vi "verify unique value in a list.vi"(7 "parameter name":string, 8 "error in (no error)":errorcluster, 9 "value":u16, 10 "list of values":u16[](array[numeric]), 11 "Simulated_CCD_Camera in":refnum<class "Simulated_CCD_Camera.lvclass">) -> (0 "error out":errorcluster, 3 "Simulated_CCD_Camera out":refnum<class "Simulated_CCD_Camera.lvclass">)   [LabVIEW 2018, in "Simulated_CCD_Camera.lvclass"]
uses:
  Simulated_CCD_Camera.lvclass
  Simulated_CCD_Camera.lvclass/Simulated_CCD_Camera.ctl
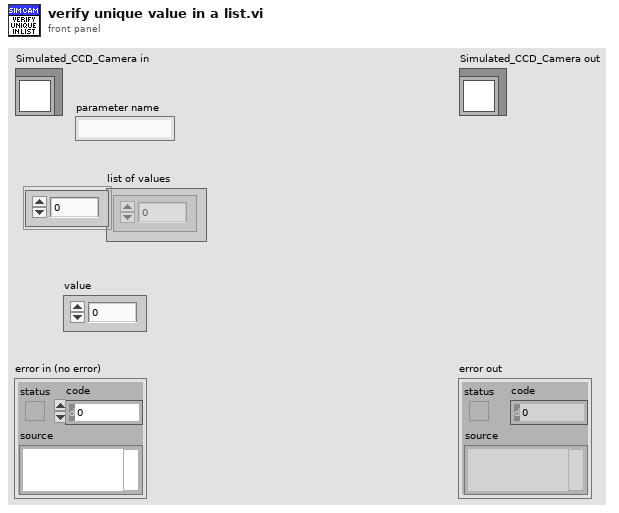
[diagram p1: front panel]
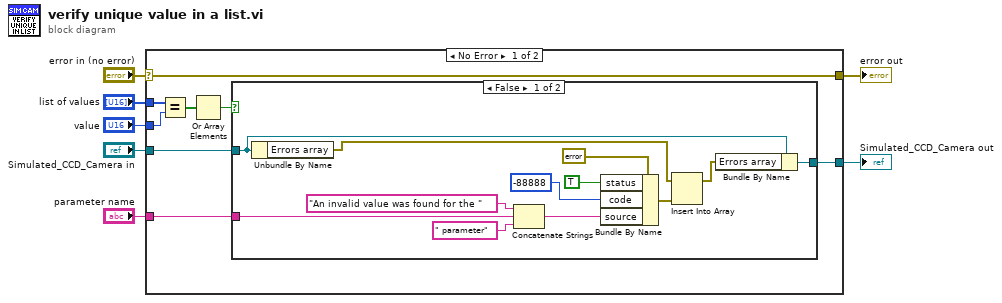
[diagram p0: block diagram]
diagram:
  n1 = case shown="No Error" "error in (no error)" {
    selector: "error in (no error)" -> [w15 w30]
    tunnel: [w15 w30] -> w6
    tunnel: [w9 w29] -> w4
    tunnel: "Simulated_CCD_Camera in" -> [w10 w29]
    tunnel: "list of values" -> [w14 _]
    tunnel: "value" -> [w13 _]
    tunnel: "parameter name" -> [w8 _]
    frame No Error {
      n2 = Equal?(x=w14, y=w13) -> (x = y?=w12:bool[])
      n3 = Or Array Elements(Boolean array=w12) -> (logical OR=w11:bool)
      n4 = case shown="False" w11 {
        tunnel: w10 -> [w24 w28]
        tunnel: [w27 w28] -> w9
        tunnel: w8 -> [w18 _]
        frame False {
          n5 = Unbundle By Name(w24) -> ("Errors array"=w26:errorcluster[])
          n6 = Concatenate Strings("An invalid value was found for the " ("source"), w18, " parameter" ("string")) -> (w16:string)
          n7 = Bundle By Name(cluster=errorcluster {"status"=FALSE, "code"=0, "source"=""} ("error constant"), "status"=TRUE, "code"=-88888, "source"=w16) -> (w20:errorcluster)
          n8 = Insert Into Array(array=w26, new element=w20) -> (w25:errorcluster[])  [unwired: 1 in]
          n9 = Bundle By Name(cluster=w24, "Errors array"=w25) -> (w27:refnum<class "Simulated_CCD_Camera.lvclass">)
        }
        frame True {
        }
      }
    }
    frame Error {
    }
  }
  "error out" <- w6
  "Simulated_CCD_Camera out" <- w4
